vi "Get Element List.vi"(8 "error in":errorcluster, 11 "Device In":T2) -> (0 "error out":errorcluster, 1 "value":T1(array[cluster]), 2 "Comm":T3, 3 "Device Out":T2)   [LabVIEW 2019]
uses:
  <userlib>/IoT Devices/_subVIs/HTTPComm.ctl
  Cluster.ctl
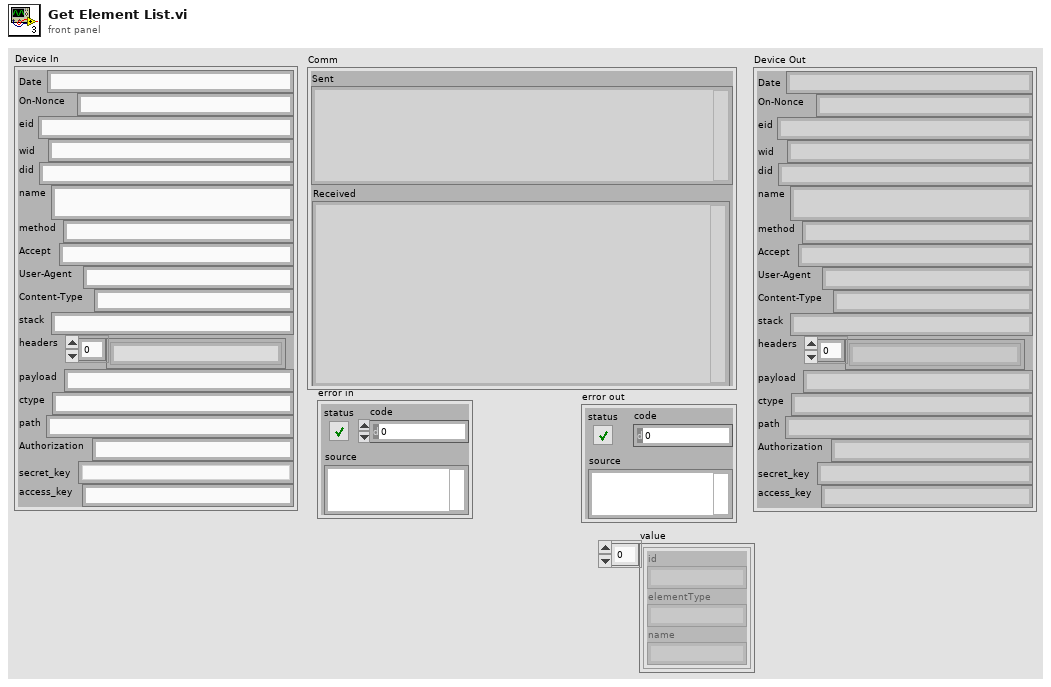
[diagram p1: front panel]
types:
  T1 = cluster{"id":string, "elementType":string, "name":string}[]
  T2 = typedef "Cluster.ctl" = cluster{"Date":string, "On-Nonce":string, "eid":string, "wid":string, "did":string, "name":string, "method":string, "Accept":string, "User-Agent":string, "Content-Type":string, "stack":string, "headers":string[], "payload":string, "ctype":string, "path":string, "Authorization":string, "secret_key":string, "access_key":string}
  T3 = typedef "HTTPComm.ctl" = cluster{"url":string, "sent headers":string, "sent body":string, "headers":string, "body":string, "Sent":string, "Received":string}
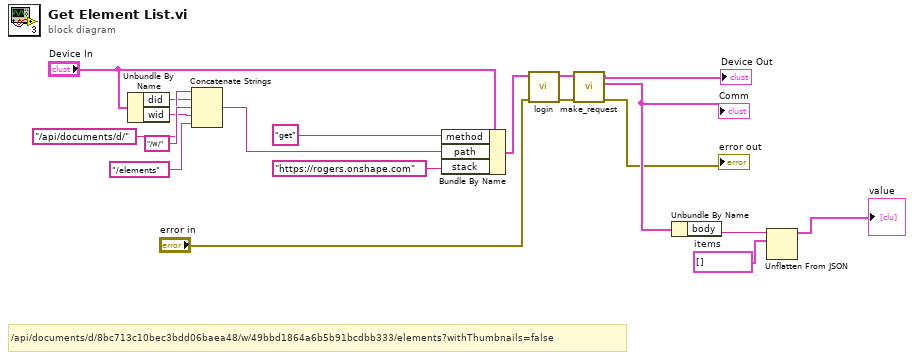
[diagram p0: block diagram]
diagram:
  w2 = T1 []  # items
  # "/api/documents/d/8bc713c10bec3bdd06baea48/w/49bbd1864a6b5b91bcdbb333/elements?withThumbnails=false"
  n1 = Unbundle By Name("Device In") -> ("did"=w6:string, "wid"=w5:string)
  n2 = Concatenate Strings("/api/documents/d/" ("payload"), w6, "/w/" ("string"), w5, "/elements" ("string")) -> (w8:string)
  n3 = Bundle By Name(cluster="Device In", "method"="get" ("Method"), "path"=w8, "stack"="https://rogers.onshape.com" ("stacks")) -> (w13:T2)
  n4 = call "login.vi"("error in"="error in", "Device In"=w13) -> ("error out"=w14:errorcluster, "Device Out"=w12:T2)  [unwired: 8 in]
  n5 = call "make_request.vi"("Error in"=w14, "Device In"=w12) -> ("error out"=→"error out":errorcluster, "Comm"=w16:T3, "Device Out"=→"Device Out":T2)  [unwired: 7 in]
  "Comm" <- w16
  n6 = Unbundle By Name(w16) -> ("body"=w3:string)
  n7 = Unflatten From JSON(JSON string=w3, type and defaults=w2) -> (value=→"value":T1)  [unwired: 5 in, 1 out]
